vi "splash.vi"() -> ()   [LabVIEW 2020, in "Volatus.lvlib" / "Plugin Splash.lvclass"]
uses:
  Plugin Splash.lvclass
panel:
  out "Version":string
  out "Status":string
  # "VOLATUS"
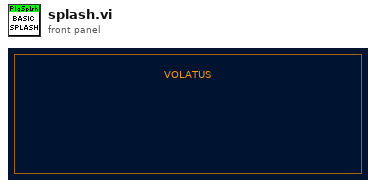
[diagram p1: front panel]
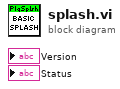
[diagram p0: block diagram]
diagram:
